vi "Split hall file.vi"(7 "name of subsetfile":path, 8 "error in":errorcluster, 9 "Length":i32, 10 "Start Index":i32, 11 "File Path":path=path "\\\\myhome\\NHMFL/Projects/Pressure/Code/Alex/m005_092123.tdms") -> (0 "error out":errorcluster)   [LabVIEW 2023]
panel:
  in  "group name in":string="p"
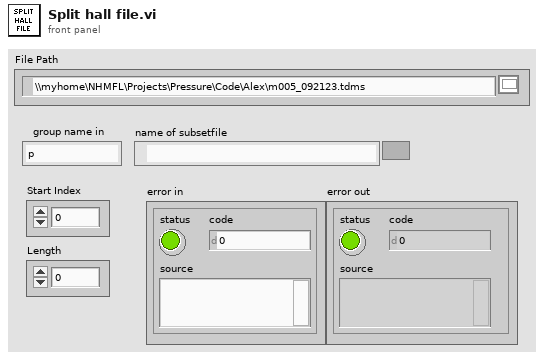
[diagram p1: front panel]
types:
  T1 = enum16{"open", "open or create", "create or replace", "create", "open (read-only)"}
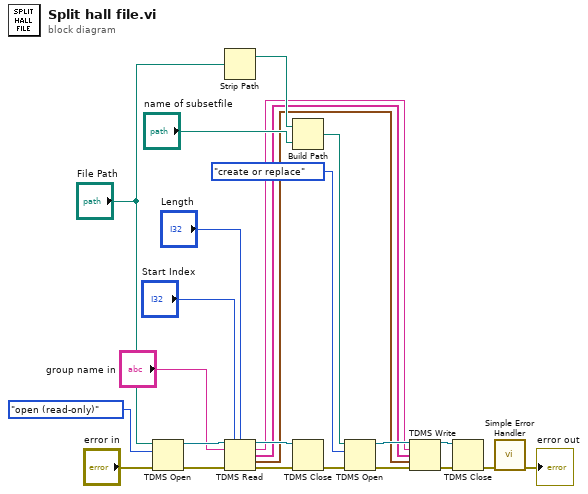
[diagram p0: block diagram]
diagram:
  n1 = TDMS Open(8:"error in", 10:T1."open (read-only)" ("operation (0:open)"), 11:"File Path") -> (0:w22:errorcluster, 3:w23:refnum<k34>)  [unwired: 4 in]
  n2 = Strip Path(path="File Path") -> (stripped path=w17:path)  [unwired: 1 out]
  n3 = TDMS Read(0:w23, 1:"Start Index", 2:"Length", 5:"group name in", 11:w22) -> (4:w20:refnum<k34>, 6:w11:string, 8:w12:string[], 10:w4:waveform(dbl)[], 15:w19:errorcluster)  [unwired: 3 in, 1 out]
  n4 = Build Path(base path=w17, name or relative path="name of subsetfile") -> (appended path=w15:path)
  n5 = TDMS Close(8:w19, 11:w20) -> (0:w10:errorcluster)  [unwired: 1 out]
  n6 = TDMS Open(8:w10, 10:T1."create or replace" ("operation (0:open)"), 11:w15) -> (0:w9:errorcluster, 3:w13:refnum<k34>)  [unwired: 4 in]
  n7 = TDMS Write(0:w13, 5:w11, 7:w12, 9:w4, 11:w9) -> (4:w8:refnum<k34>, 15:w7:errorcluster)  [unwired: 1 in, 2 out]
  n8 = TDMS Close(8:w7, 11:w8) -> (0:w1:errorcluster)  [unwired: 1 out]
  n9 = call <vilib>:"Simple Error Handler.vi"("error in (no error)"=w1) -> ("error out"=→"error out":errorcluster)  [unwired: 4 in, 4 out]
